vi "VolltagePeltierResonanceCurve.vi"(2 "TemperatureError":dbl=200.0 format="%.2f", 3 "Temperature":dbl=200.0 format="%.2f", 5 "#Measurements each Frequency":i32=200, 6 "Step":dbl=200.0 format="%.2f", 8 "error in":errorcluster, 9 "Stop":dbl=200.0 format="%.2f", 10 "Start":dbl=200.0 format="%.2f", 11 "Voltage":dbl=200.0 format="%.2f") -> (0 "error out":errorcluster)   [LabVIEW 2010]
panel:
  in  "Path":path
  in  "Wait":dbl=200.0 format="%.2f"
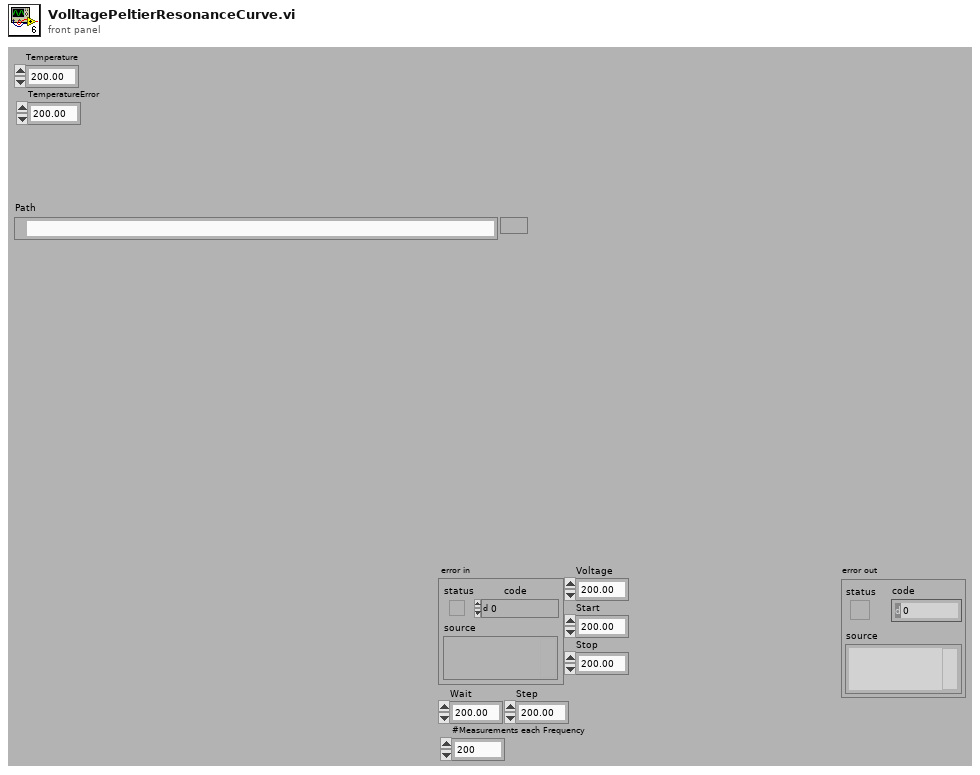
[diagram p1: front panel]
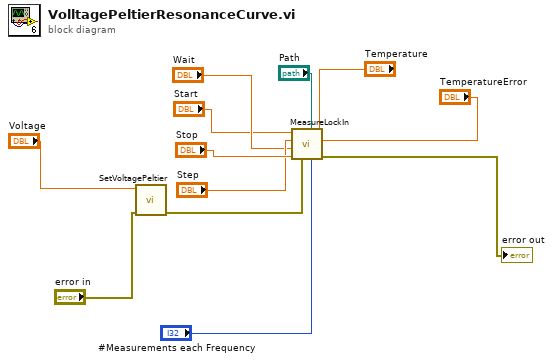
[diagram p0: block diagram]
diagram:
  n1 = call "SetVoltagePeltier.vi"("error in"="error in", "Voltage"="Voltage") -> ("error out"=w5:errorcluster)  [unwired: 9 in]
  n2 = call "MeasureLockIn.vi"("TemperatureError"="TemperatureError", "Temperature"="Temperature", "#Measurements each Frequency"="#Measurements each Frequency", "Path"="Path", "error in"=w5, "Stop"="Stop", "Wait (ms)"="Wait", "Step"="Step", "Start"="Start") -> ("error out"=→"error out":errorcluster)  [unwired: 2 in]
